vi "SLSC Show Pinout.vi"(9 "Type":string="_pinout.png", 10 "number":i32, 11 "Vendor Name":string) -> ()   [LabVIEW 2020, in "SLSC EDS System Explorer.lvlib"]
uses:
  SLSC EDS System Explorer.lvlib
panel:
  out "2D Picture":picture
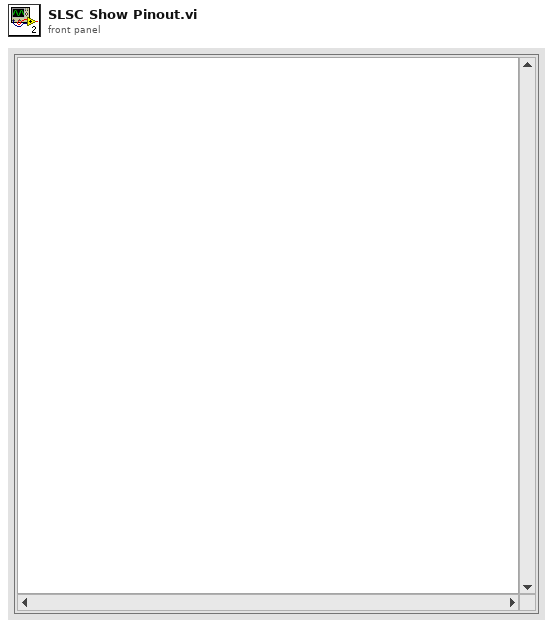
[diagram p1: front panel]
types:
  T1 = typedef "imagedata.ctl" = cluster{"image type":i32, "image depth":i32, "image":u8[], "mask":u8[], "colors":u32[], "Rectangle":cluster{"left":i16, "top":i16, "right":i16, "bottom":i16}}
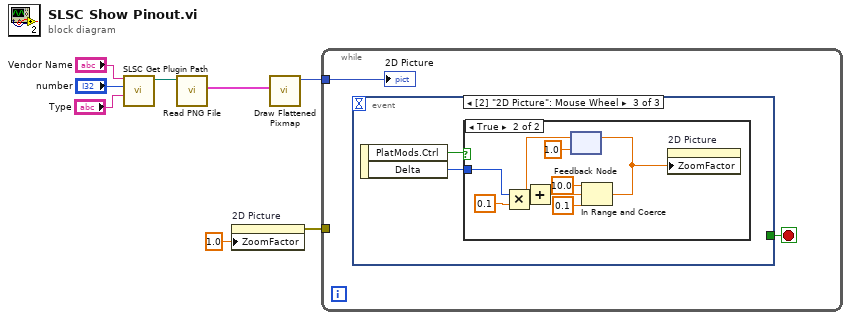
[diagram p0: block diagram]
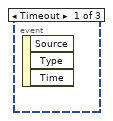
[diagram p2: hidden frame]
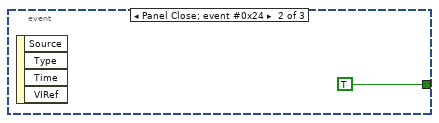
[diagram p3: hidden frame]
diagram:
  n1 = call "SLSC Get Plugin Path.vi"("Type"="Type", "number"="number", "Vendor Prefix"="Vendor Name") -> ("appended path"=w4:path)  [unwired: 8 in]
  n2 = call <vilib>:"Read PNG File.vi"("path to PNG file"=w4) -> ("image data"=w8:T1)  [unwired: 8 in, 2 out]
  n3 = property on="2D Picture" class="Pict"("ZoomFactor"=sgl 1.0 ("Zoom Factor")) -> (error out=w5:errorcluster)  [unwired: 2 in, 1 out]
  n4 = call <vilib>:"Draw Flattened Pixmap.vi"("image data"=w8) -> ("new picture"=w7:picture)  [unwired: 8 in]
  n5 = while {
    tunnel: w7 -> [w9]
    tunnel: w5 -> [_]
    stop <- w10 stop-if-true
    n6 = event shown="[2] \"2D Picture\": Mouse Wheel" {
      selector: _ -> [_ _ _]
      dyn-events: _ -> [_ _ _]
      timeout: _ -> [_ _ _]
      tunnel: [_ TRUE _] -> w10
      event Timeout {
        n7 = event-data() -> ()  [unwired: 1 in, 3 out]
      }
      event Panel Close; event #0x24 {
        n8 = event-data() -> ()  [unwired: 1 in, 4 out]
      }
      event "2D Picture": Mouse Wheel {
        n9 = event-data() -> ("PlatMods.Ctrl"=w12:bool, "Delta"=w13:i32)  [unwired: 1 in]
        n10 = case shown="True" w12 {
          tunnel: w13 -> [_ w18]
          frame False {
          }
          frame True {
            n11 = Multiply(x=w18, y=0.1) -> (x*y=w21:dbl)
            n12 = feedback #1(1.0 ("upper limit")) -> (w19:dbl)
            n13 = Add(x=w19, y=w21) -> (x+y=w20:dbl)
            n14 = In Range and Coerce(upper limit=10.0, x=w20, lower limit=0.1) -> (coerced(x)=w17:dbl)  [unwired: 1 out]
            n15 = feedback-in #1(w17) -> ()
            n16 = property on="2D Picture" class="Pict"("ZoomFactor"=w17) -> ()  [unwired: 2 in, 2 out]
          }
        }
      }
    }
    "2D Picture" <- w9
  }
